vi "G#Debugger_CachedObject.vi"(1 "cached object":refnum<class "G#Object.lvclass">, 5 "error in (no error)":errorcluster, 6 "set":bool) -> (15 "cached object out":refnum<class "G#Object.lvclass">, 17 "not a refnum?":bool, 19 "error out":errorcluster)   [LabVIEW 2017, in "G#Debugger.lvlib"]
doc: "Caches an instance of the last created debugger object in active debug mode."
uses:
  G#Debugger.lvlib
  G#Object/G#Object.lvclass
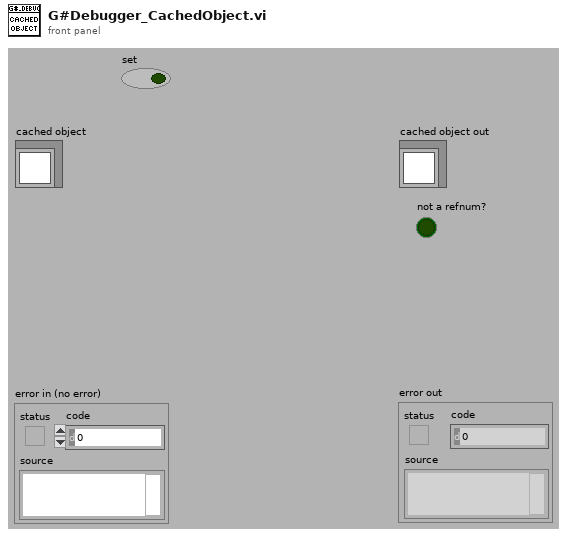
[diagram p1: front panel]
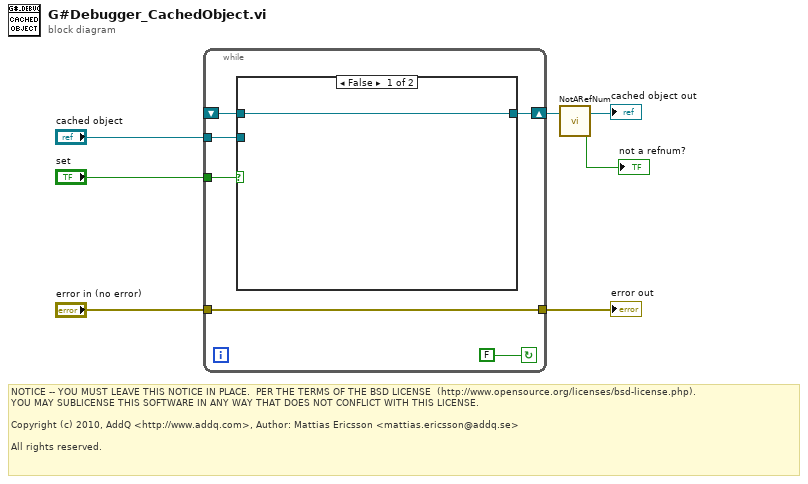
[diagram p0: block diagram]
diagram:
  # "NOTICE -- YOU MUST LEAVE THIS NOTICE IN PLACE.  PER THE TERMS OF THE BSD LICENSE  (http://www.opensource.org/licenses/bsd-license.php).\nYOU MAY SUBLICENSE THIS SOFTWARE IN ANY WAY THAT DOES NOT CONFLICT WITH THIS LICENSE.\n\nCopyright (c) 2010, AddQ <http://www.addq.com>, Author: Mattias Ericsson <mattias.ericsson@addq.se>\n\nAll rights reserved."
  n1 = while {
    tunnel: "error in (no error)" -> [w12]
    tunnel: [w12] -> w6
    tunnel: "set" -> [w11]
    shift-right: [w10] -> w3
    shift-left: _ -> [w8]
    tunnel: "cached object" -> [w9]
    stop <- FALSE continue-if-true
    n2 = case shown="False" w11 {
      tunnel: [w14 w15] -> w10
      tunnel: w9 -> [_ w15]
      tunnel: w8 -> [w14 _]
      frame False {
      }
      frame True {
      }
    }
  }
  "error out" <- w6
  n3 = call-dynamic "NotARefNum.vi"("reference in"=w3) -> ("not a refnum?"=→"not a refnum?":bool, "reference out"=→"cached object out":refnum<class "G#Object.lvclass">)  [unwired: 1 in]
